vi "ReadAcquisitionBlockSize.vi"(8 "error in (no error)":errorcluster, 11 "Map":T1) -> (0 "error out":errorcluster, 2 "Found?":bool, 3 "Block Size (s)":dbl)   [LabVIEW 2017]
uses:
  <vilib>/addons/PointValueMap/controls/PointMap.ctl
  <vilib>/addons/PointValueMap/subVIs/Point_Read_double.vi
  <vilib>/addons/PointValueMap/PointValueMap.lvlib
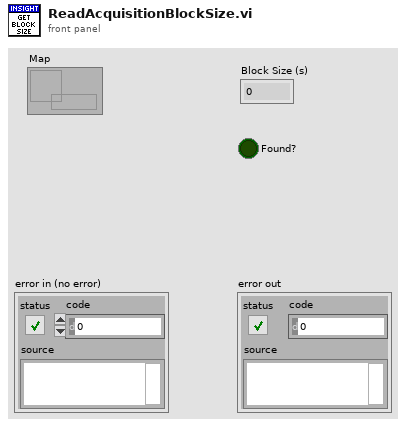
[diagram p1: front panel]
types:
  T1 = typedef "PointValueMap.lvlib/PointMap.ctl" = refnum<data-value>
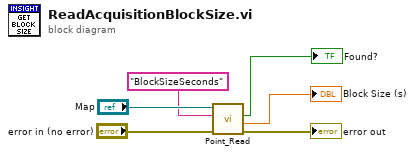
[diagram p0: block diagram]
diagram:
  n1 = call-poly <vilib>:"Point_Read.vi"("Error In"="error in (no error)", "Tag"="BlockSizeSeconds", "Map"="Map") -> ("Error Out"=→"error out":errorcluster, "Value"=→"Block Size (s)":dbl, "Found?"=→"Found?":bool)  [unwired: 3 in, 3 out]
